vi "Copy .LLB to NI VeriStand dir.vi"(5 "Files Generated by Build":path[](array[path]), 6 "Top Level/Always Included VIs":path[](array[path]), 7 "Destination Path":path, 8 "error in (no error)":errorcluster, 9 "Target Name":string, 10 "Build Specification Name":string, 11 "Project Path":path) -> (0 "error out":errorcluster)   [LabVIEW 2023, in "NI PXIe-411x PS Custom Device.lvlib"]
doc: "This VI is called after each run of a build specification. The VI will copy the generated LLB (Engine or System Explorer) into the VeriStand Custom Device folder (...\\Documents\\National Instruments\\NI VeriStand 2013...)."
uses:
  NI PXIe-411x PS Custom Device.lvlib
  <vilib>/Utility/sysdir.llb/System Directory Type.ctl
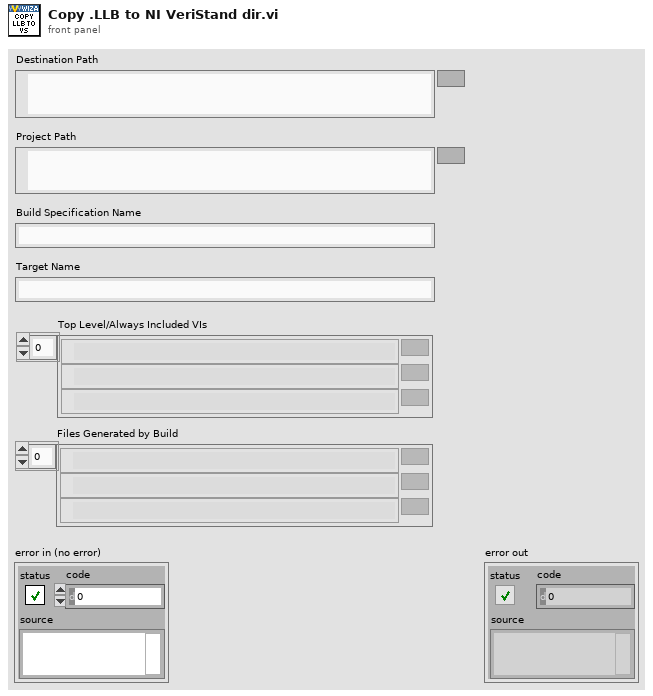
[diagram p1: front panel]
types:
  T1 = typedef "System Directory Type.ctl" = i32
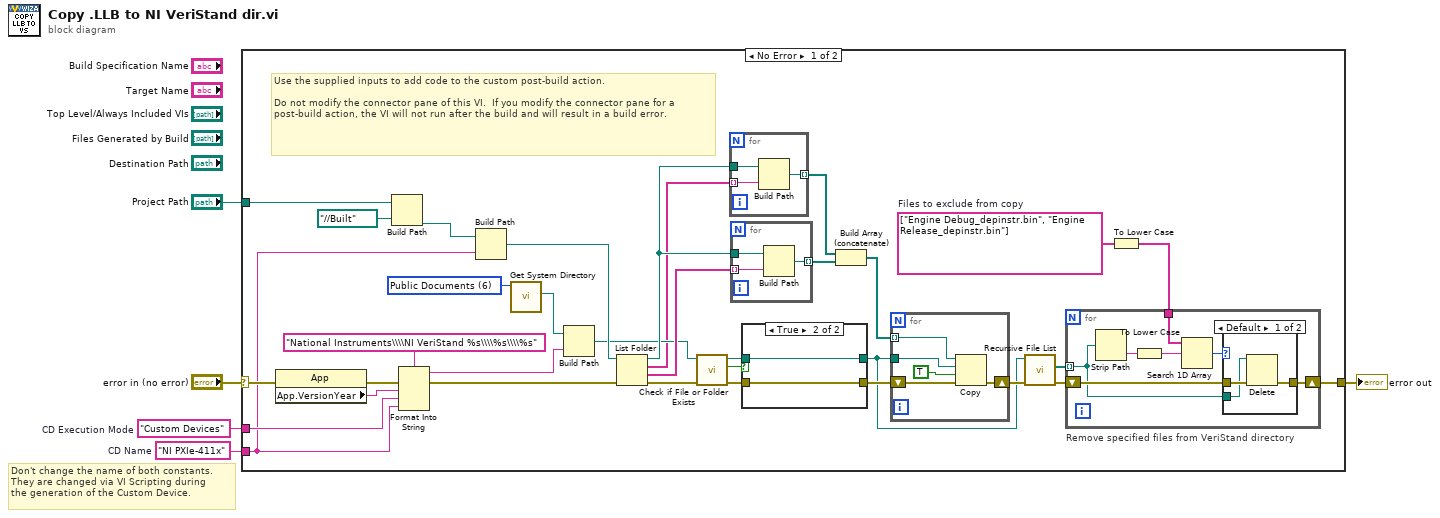
[diagram p0: block diagram]
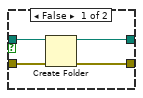
[diagram p3: hidden frame]
diagram:
  w2 = "NI PXIe-411x"  # CD Name
  w3 = "Custom Devices"  # CD Execution Mode
  # "Don't change the name of both constants.\nThey are changed via VI Scripting during\nthe generation of the Custom Device."
  n1 = case shown="No Error" "error in (no error)" {
    selector: "error in (no error)" -> [w19 w67]
    tunnel: [w6 w67] -> w1
    tunnel: "Project Path" -> [w15 _]
    tunnel: w3 -> [w20 _]
    tunnel: w2 -> [w17 _]
    frame No Error {
      w12 = string[] ["Engine Debug_depinstr.bin", "Engine Release_depinstr.bin"]  # Files to exclude from copy
      w25 = T1 6 items=["User Home"=0, "User Desktop"=1, "User Documents"=2, "User Application Data"=3, "User Preferences"=4, "User Temporary"=5, "Public Documents"=6, "Public Application Data"=7, "Public Preferences"=8, "Public Cache"=13, "System Core Libraries"=9, "System Installed Libraries"=10, "Application Files"=11, "Boot Volume Root"=12] ("system directory type")
      # "Use the supplied inputs to add code to the custom post-build action.\n\nDo not modify the connector pane of this VI.  If you modify the connector pane for a post-build action, the VI will not run after the build and will result in a build error."
      n2 = property class="App"(error in=w19) -> (error out=w24:errorcluster, "App.VersionYear"=w23:string)  [unwired: 1 in, 1 out]
      n3 = Build Path(base path=w15, name or relative path=path "../../Built") -> (appended path=w28:path)
      n4 = Format Into String(format string="National Instruments\\\\NI VeriStand %s\\\\%s\\\\%s" ("name or relative path"), error in=w24, w23, w20, w17) -> (resulting string=w27:string, error out=w18:errorcluster)  [unwired: 1 in]
      n5 = Build Path(base path=w28, name or relative path=w17) -> (appended path=w30:path)
      n6 = call <vilib>:"Get System Directory.vi"("system directory type"=w25) -> ("system directory"=w26:path)  [unwired: 10 in]
      n7 = Build Path(base path=w26, name or relative path=w27) -> (appended path=w21:path)
      n8 = List Folder(path=w30, error in=w18) -> (path out=w32:path, filenames=w13:string[], folder names=w33:string[], error out=w29:errorcluster)  [unwired: 2 in]
      n9 = call <vilib>:"Check if File or Folder Exists.vi"("error in (no error)"=w29, "path"=w21) -> ("error out"=w34:errorcluster, "file or folder exists?"=w36:bool, "dup path"=w35:path)  [unwired: 7 in]
      n10 = for {
        tunnel: w13 -> [w65] mode=indexing
        tunnel: w32 -> [w66]
        tunnel: [w64] -> w38 mode=indexing
        n11 = Build Path(base path=w66, name or relative path=w65) -> (appended path=w64:path)
      }
      n12 = for {
        tunnel: w33 -> [w62] mode=indexing
        tunnel: w32 -> [w63]
        tunnel: [w61] -> w31 mode=indexing
        n13 = Build Path(base path=w63, name or relative path=w62) -> (appended path=w61:path)
      }
      n14 = case shown="True" w36 {
        tunnel: w35 -> [w53 w55]
        tunnel: w34 -> [w52 w54]
        tunnel: [w51 w55] -> w7
        tunnel: [w50 w54] -> w14
        frame False {
          n15 = Create Folder(path (use dialog)=w53, error in=w52) -> (created path=w51:path, error out=w50:errorcluster)  [unwired: 1 in, 1 out]
        }
        frame True {
        }
      }
      n16 = Build Array (concatenate)(w38, w31) -> (w37:path[])
      n17 = for {
        tunnel: w37 -> [w57] mode=indexing
        shift-right: [w58] -> w8
        shift-left: w14 -> [w59]
        tunnel: w7 -> [w56]
        n18 = Copy(8:w59, 9:TRUE ("overwrite (F)"), 10:w56, 11:w57) -> (0:w58:errorcluster)  [unwired: 1 in, 2 out]
      }
      n19 = call <vilib>:"Recursive File List.vi"("error in (no error)"=w8, "Folder Path"=w7) -> ("error out"=w11:errorcluster, "All Files in Dir"=w10:path[])  [unwired: 5 in, 3 out]
      n20 = To Lower Case(string=w12) -> (all lower case string=w9:string[])
      n21 = for "Remove specified files from VeriStand directory" {
        shift-right: [w40] -> w6
        shift-left: w11 -> [w42]
        tunnel: w10 -> [w39] mode=indexing
        tunnel: w9 -> [w43]
        n22 = Strip Path(path=w39) -> (name=w45:string)  [unwired: 1 out]
        n23 = To Lower Case(string=w45) -> (all lower case string=w44:string)
        n24 = Search 1D Array(1D array=w43, element=w44) -> (index of element=w41:i32)  [unwired: 1 in]
        n25 = case shown="Default" w41 {
          tunnel: w42 -> [w48 w49]
          tunnel: [w47 w49] -> w40
          tunnel: w39 -> [w46 _]
          frame Default {
            n26 = Delete(path (use dialog)=w46, error in=w48) -> (error out=w47:errorcluster)  [unwired: 3 in, 2 out]
          }
          frame -1 {
          }
        }
      }
    }
    frame Error {
    }
  }
  "error out" <- w1
